vi "Analog Out Scan.vi"(8 "error in (no error)":errorcluster, 11 "Analog Out Scan in":refnum<class "Analog Out Scan.lvclass">) -> (0 "error out":errorcluster, 3 "Analog Out Scan out":refnum<class "Analog Out Scan.lvclass">)   [LabVIEW 2009, in "Analog Out Scan.lvclass"]
uses:
  Analog Out Scan.lvclass
  Scanner/Scanner.lvclass
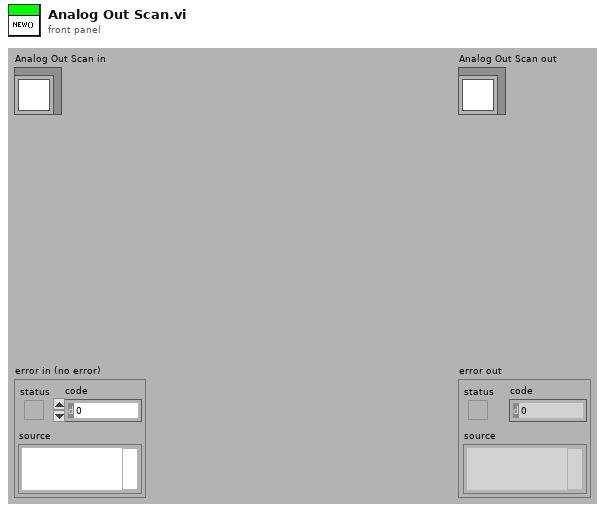
[diagram p1: front panel]
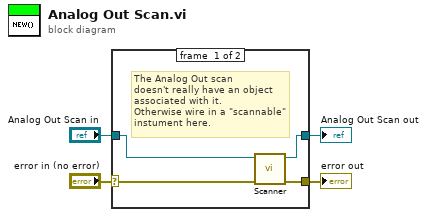
[diagram p0: block diagram]
diagram:
  n1 = case shown="No Error" "error in (no error)" {
    selector: "error in (no error)" -> [w6 w10]
    tunnel: [w5 w10] -> w3
    tunnel: [w7 w9] -> w1
    tunnel: "Analog Out Scan in" -> [w8 w9]
    frame #0 {
      # "The Analog Out scan \ndoesn't really have an object\nassociated with it.\nOtherwise wire in a \"scannable\" \ninstument here."
      n2 = call "Scanner.vi"("error in (no error)"=w6, "Scanner.lvclass in"=w8) -> ("error out"=w5:errorcluster, "Scanner.lvclass out"=w7:refnum<class "Analog Out Scan.lvclass">)  [unwired: 2 in, 6 out]
    }
    frame #1 {
    }
  }
  "error out" <- w3
  "Analog Out Scan out" <- w1
